vi "Run.vi"(8 "error in (no error)":errorcluster, 11 "SPARC4_GUI in":refnum<class "SPARC4_GEI.lvclass">) -> (0 "error out":errorcluster, 3 "SPARC4_GUI out":refnum<class "SPARC4_GEI.lvclass">)   [LabVIEW 2018, in "SPARC4_GEI.lvclass"]
uses:
  SPARC4_GEI.lvclass
  SPARC4_GEI.lvclass/SPARC4_GEI.ctl
  Channel GUI/Channel GEI.lvclass
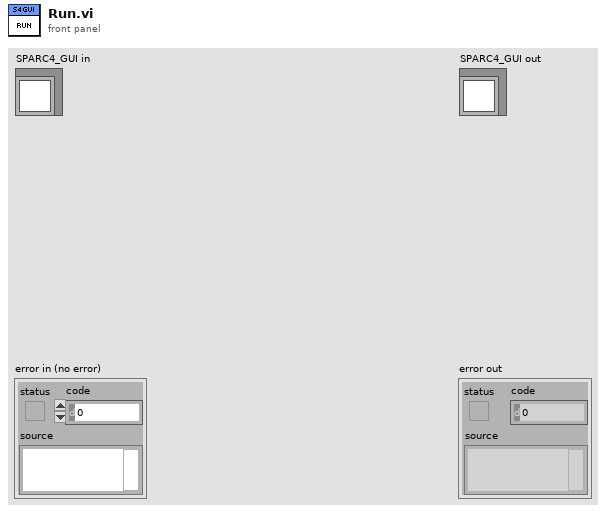
[diagram p1: front panel]
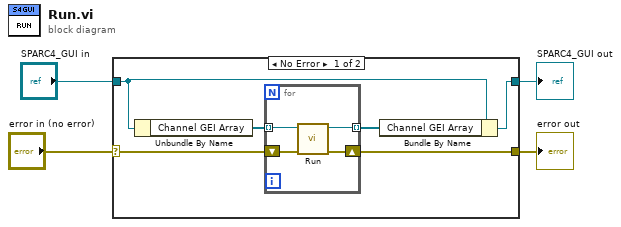
[diagram p0: block diagram]
diagram:
  n1 = case shown="No Error" "error in (no error)" {
    selector: "error in (no error)" -> [w9 w16]
    tunnel: [w8 w16] -> w3
    tunnel: [w5 w15] -> w1
    tunnel: "SPARC4_GUI in" -> [w7 w15]
    frame No Error {
      n2 = Unbundle By Name(w7) -> ("Channel GEI Array"=w10:refnum<class "Channel GEI.lvclass">[])
      n3 = for {
        tunnel: w10 -> [w14] mode=indexing
        tunnel: [w12] -> w6 mode=indexing
        shift-right: [w11] -> w8
        shift-left: w9 -> [w13]
        n4 = call "Run.vi"("error in (no error)"=w13, "Channel GUI in"=w14) -> ("error out"=w11:errorcluster, "Channel GUI out"=w12:refnum<class "Channel GEI.lvclass">)  [unwired: 8 in]
      }
      n5 = Bundle By Name(cluster=w7, "Channel GEI Array"=w6) -> (w5:refnum<class "SPARC4_GEI.lvclass">)
    }
    frame Error {
    }
  }
  "error out" <- w3
  "SPARC4_GUI out" <- w1
